vi "DBVar TriggeredByType.vi"(1 "data classification":T1(ring), 2 "type  classification":T2(ring), 3 "type not equal?":bool) -> (0 "Trigger?":bool)   [LabVIEW 2020, in "NI_DB Variant To Data Support.lvlib"]
uses:
  <vilib>/addons/database/_DB Variant To Data/NI_DB Variant To Data Support.lvlib
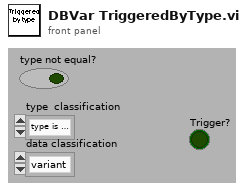
[diagram p1: front panel]
types:
  T1 = enum16{"variant", "variant 1D array", "variant 2D array", "others"}
  T2 = enum16{"type is cluster", "type is 1D array of scalar type", "type is 1D array of cluster type", "type is 2D array", "type is others", "type is unwired"}
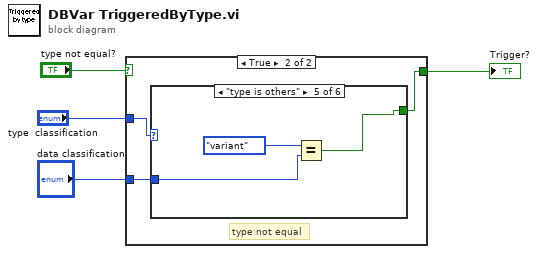
[diagram p0: block diagram]
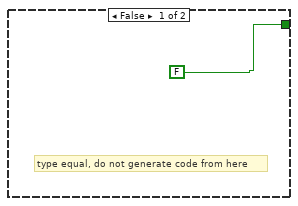
[diagram p2: hidden frame]
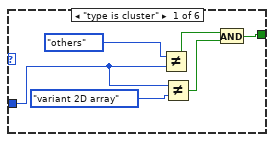
[diagram p3: hidden frame]
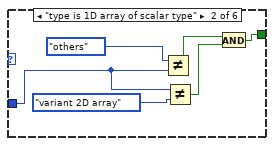
[diagram p4: hidden frame]
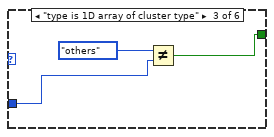
[diagram p5: hidden frame]
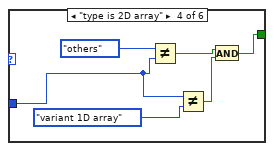
[diagram p6: hidden frame]
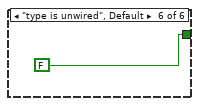
[diagram p7: hidden frame]
diagram:
  n1 = case shown="True" "type not equal?" {
    tunnel: [FALSE w7] -> w1
    tunnel: "data classification" -> [_ w8]
    tunnel: "type  classification" -> [_ w6]
    frame False {
      # "type equal, do not generate code from here"
    }
    frame True {
      # "type not equal"
      n2 = case shown="\"type is others\"" w6 {
        tunnel: w8 -> [w9 w15 w22 w27 w31 _]
        tunnel: [w10 w18 w21 w26 w30 FALSE] -> w7
        frame "type is cluster" {
          n3 = Not Equal?(x=T1."others" ("GenData"), y=w9) -> (x != y?=w12:bool)
          n4 = Not Equal?(x=w9, y=T1."variant 2D array" ("GenData")) -> (x != y?=w11:bool)
          n5 = And(x=w12, y=w11) -> (x .and. y?=w10:bool)
        }
        frame "type is 1D array of scalar type" {
          n6 = Not Equal?(x=T1."others" ("GenData"), y=w15) -> (x != y?=w17:bool)
          n7 = Not Equal?(x=w15, y=T1."variant 2D array" ("GenData")) -> (x != y?=w16:bool)
          n8 = And(x=w17, y=w16) -> (x .and. y?=w18:bool)
        }
        frame "type is 1D array of cluster type" {
          n9 = Not Equal?(x=T1."others" ("GenData"), y=w22) -> (x != y?=w21:bool)
        }
        frame "type is 2D array" {
          n10 = Not Equal?(x=T1."others" ("GenData"), y=w27) -> (x != y?=w25:bool)
          n11 = Not Equal?(x=w27, y=T1."variant 1D array" ("GenData")) -> (x != y?=w24:bool)
          n12 = And(x=w25, y=w24) -> (x .and. y?=w26:bool)
        }
        frame "type is others" {
          n13 = Equal?(x=T1."variant" ("GenData"), y=w31) -> (x = y?=w30:bool)
        }
        frame "type is unwired", Default {
        }
      }
    }
  }
  "Trigger?" <- w1
